vi "Class XML FGV.vi"(6 "Function":enum16{"read", "write"}(ring), 8 "error in (no error)":errorcluster, 11 "LabVIEW Object":refnum<class>) -> (0 "error out":errorcluster, 3 "Control Experiment.lvclass out":refnum<class>)   [LabVIEW 2019, in "SMO.Control Experiment.lvclass"]
uses:
  SMO.Control Experiment.lvclass
  <vilib>/Utility/sysdir.llb/System Directory Type.ctl
  <vilib>/Utility/xml.llb/Write to XML File(string).vi
  <vilib>/Utility/xml.llb/Read From XML File(string).vi
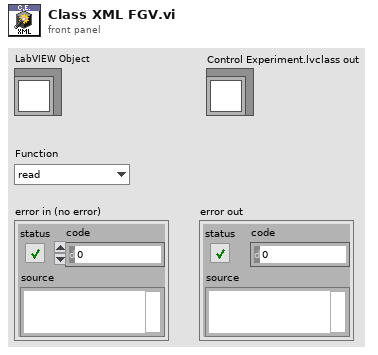
[diagram p1: front panel]
types:
  T1 = typedef "System Directory Type.ctl" = i32
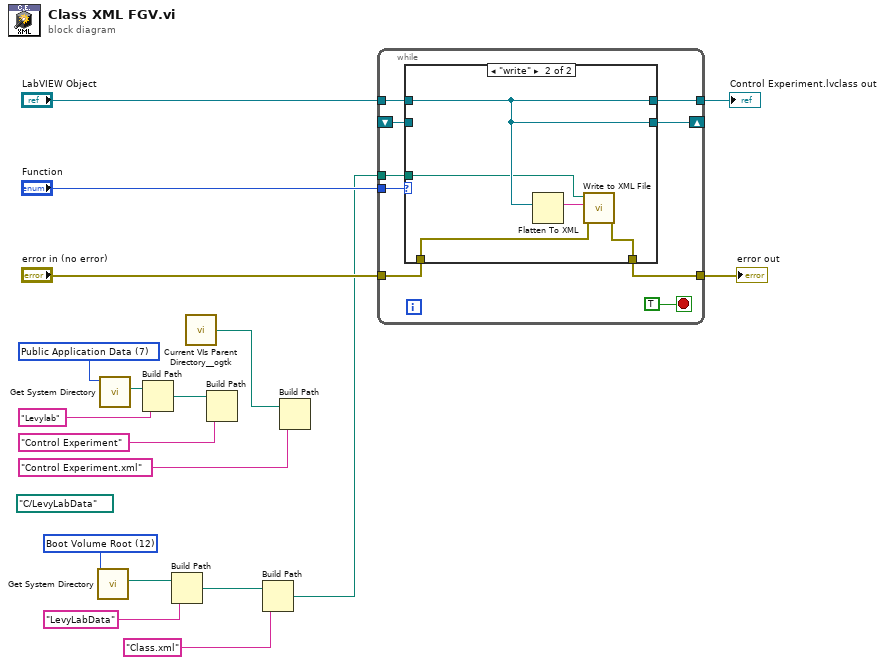
[diagram p0: block diagram]
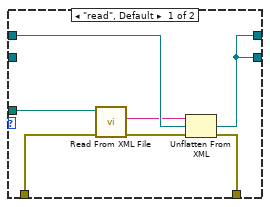
[diagram p2: hidden frame]
diagram:
  w6 = T1 12 items=["User Home"=0, "User Desktop"=1, "User Documents"=2, "User Application Data"=3, "User Preferences"=4, "User Temporary"=5, "Public Documents"=6, "Public Application Data"=7, "Public Preferences"=8, "Public Cache"=13, "System Core Libraries"=9, "System Installed Libraries"=10, "Application Files"=11, "Boot Volume Root"=12] ("system directory type")
  (unwired) path "C:/LevyLabData" ("Directory Path")
  w12 = T1 7 items=["User Home"=0, "User Desktop"=1, "User Documents"=2, "User Application Data"=3, "User Preferences"=4, "User Temporary"=5, "Public Documents"=6, "Public Application Data"=7, "Public Preferences"=8, "Public Cache"=13, "System Core Libraries"=9, "System Installed Libraries"=10, "Application Files"=11, "Boot Volume Root"=12] ("system directory type")
  n1 = call <vilib>:"Get System Directory.vi"("system directory type"=w6) -> ("system directory"=w5:path)  [unwired: 10 in]
  n2 = call <vilib>:"Get System Directory.vi"("system directory type"=w12) -> ("system directory"=w9:path)  [unwired: 10 in]
  n3 = Build Path(base path=w9, name or relative path="Levylab") -> (appended path=w11:path)
  n4 = Build Path(base path=w5, name or relative path="LevyLabData") -> (appended path=w3:path)
  n5 = call <userlib>:"Current VIs Parent Directory__ogtk.vi"() -> ("Parent Directory (+ Relative)"=w7:path)  [unwired: 5 in]
  n6 = Build Path(base path=w11, name or relative path="Control Experiment") -> ()  [unwired: 1 out]
  n7 = Build Path(base path=w3, name or relative path="Class.xml") -> (appended path=w1:path)
  n8 = Build Path(base path=w7, name or relative path="Control Experiment.xml") -> ()  [unwired: 1 out]
  n9 = while {
    tunnel: "LabVIEW Object" -> [w24]
    tunnel: "error in (no error)" -> [w21]
    tunnel: [w20] -> w18
    tunnel: [w23] -> w14
    shift-right: [w25] -> _
    shift-left: _ -> [w22]
    tunnel: "Function" -> [w26]
    tunnel: w1 -> [w19]
    stop <- TRUE stop-if-true
    n10 = case shown="\"write\"" w26 {
      tunnel: [w33 w39] -> w25
      tunnel: w24 -> [w32 w39]
      tunnel: [w33 w39] -> w23
      tunnel: w22 -> [_ _]
      tunnel: w21 -> [w29 w38]
      tunnel: [w34 w35] -> w20
      tunnel: w19 -> [w31 w36]
      frame "read", Default {
        n11 = call-poly <vilib>:"Read From XML File.vi"("error in (no error)"=w29, "XML File Path"=w31) -> ("error out"=w28:errorcluster, "XML Elements"=w30:string)  [unwired: 7 in, 1 out]
        n12 = Unflatten From XML(xml string=w30, type=w32, error in (no error)=w28) -> (value=w33:refnum<class>, error out=w34:errorcluster)
      }
      frame "write" {
        n13 = Flatten To XML(anything=w39) -> (xml string=w37:string)
        n14 = call-poly <vilib>:"Write to XML File.vi"("error in (no error)"=w38, "XML Input"=w37, "XML File Path"=w36) -> ("error out"=w35:errorcluster)  [unwired: 6 in, 2 out]
      }
    }
  }
  "error out" <- w18
  "Control Experiment.lvclass out" <- w14
